vi "DB Tools Get Properties.vi"   [LabVIEW 2020, in "NI_Database_API.lvlib"]
doc: "Gets properties of the object as determined by the inputs. This VI works for connections, commands, recordsets, columns, and parameters. Wire data to the reference input to determine the polymorphic instance to use or manually select the instance."
uses:
  <vilib>/addons/database/NI_Database_API.lvlib
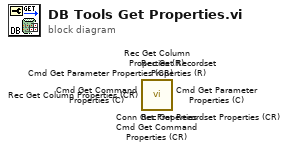
[diagram p0: block diagram]
diagram:
  n1 = call <vilib>:"Conn Get Properties.vi"() -> ()  [unwired: 5 in, 3 out]
  n2 = call <vilib>:"Rec Get Recordset Properties (R).vi"() -> ()  [unwired: 5 in, 3 out]
  n3 = call <vilib>:"Cmd Get Command Properties (C).vi"() -> ()  [unwired: 5 in, 3 out]
  n4 = call <vilib>:"Cmd Get Parameter Properties (C).vi"() -> ()  [unwired: 5 in, 3 out]
  n5 = call <vilib>:"Cmd Get Command Properties (CR).vi"() -> ()  [unwired: 5 in, 3 out]
  n6 = call <vilib>:"Cmd Get Parameter Properties (CR).vi"() -> ()  [unwired: 5 in, 3 out]
  n7 = call <vilib>:"Rec Get Column Properties (R).vi"() -> ()  [unwired: 5 in, 3 out]
  n8 = call <vilib>:"Rec Get Recordset Properties (CR).vi"() -> ()  [unwired: 5 in, 3 out]
  n9 = call <vilib>:"Rec Get Column Properties (CR).vi"() -> ()  [unwired: 5 in, 3 out]
